vi "Send Command.vi"(6 "Command":T1, 8 "error in":errorcluster, 10 "Value":dbl, 11 "Thorlabs In":refnum<class "Thorlabs.lvclass">) -> (0 "error out":errorcluster, 3 "Thorlabs Out":refnum<class "Thorlabs.lvclass">)   [LabVIEW 2018, in "Thorlabs.lvlib" / "Thorlabs.lvclass"]
doc: "This VI is designed to take in all the possible Commands, and perform the proper functions of that Command. If the Command is not supported nothing happens.\n\nCreator: Slade Jeppesen\nCreated Date: 09/29/20"
uses:
  Thorlabs.lvclass
  PPLs/Axis/Parent/Axis.lvlibp/Custom Controls/Command.ctl
  PPLs/Axis/Parent/Axis.lvlibp
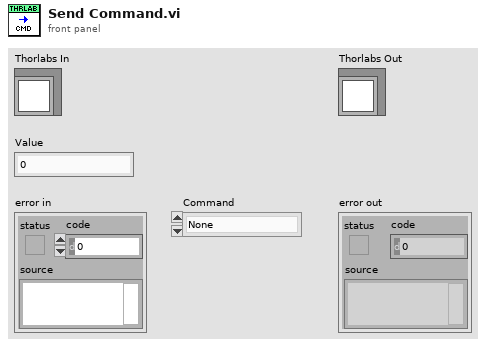
[diagram p1: front panel]
types:
  T1 = typedef "Axis.lvlibp/Command.ctl" = enum16{"None", "Home", "Renumber", "Move Absolute", "Move Relative", "Stop", "Set Run Speed", "Set Acceleration", "Set Run Current", "Set Home Offset", "Set Home Speed", "Query Current Position", "Load Defaults", "Query Status", "Lock Controls", "Unlock Controls", "Set Jog Step Size", "Set Jog Acceleration", "Set Jog Speed", "Query Homed Status", "Query Moving Status", "Reset", "Set Max Position", "Set Min Position"}
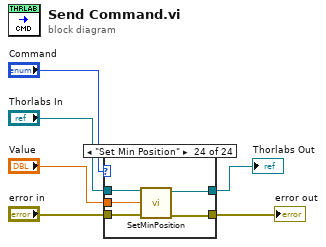
[diagram p0: block diagram]
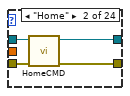
[diagram p3: hidden frame]
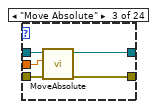
[diagram p4: hidden frame]
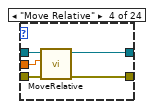
[diagram p5: hidden frame]
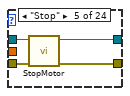
[diagram p6: hidden frame]
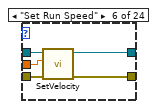
[diagram p7: hidden frame]
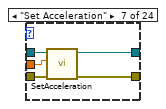
[diagram p8: hidden frame]
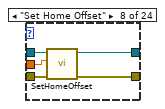
[diagram p9: hidden frame]
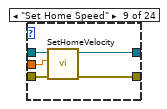
[diagram p10: hidden frame]
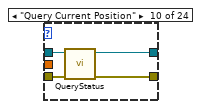
[diagram p11: hidden frame]
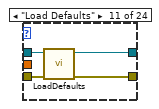
[diagram p12: hidden frame]
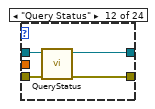
[diagram p13: hidden frame]
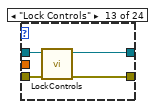
[diagram p14: hidden frame]
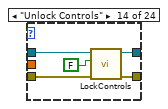
[diagram p15: hidden frame]
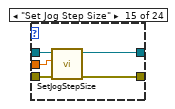
[diagram p16: hidden frame]
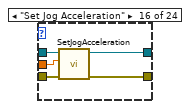
[diagram p17: hidden frame]
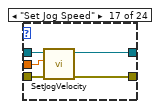
[diagram p18: hidden frame]
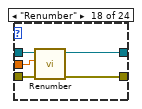
[diagram p19: hidden frame]
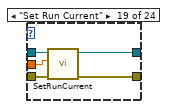
[diagram p20: hidden frame]
diagram:
  n1 = case shown="\"Set Min Position\"" "Command" {
    tunnel: "Value" -> [_ _ w16 w18 _ w30 w35 w40 w44 _ _ _ _ _ w71 w75 w80 w83 w88 _ _ _ w108 w110]
    tunnel: "Thorlabs In" -> [w7 w11 w15 w19 w25 w29 w34 w39 w45 w49 w53 w57 w61 w66 w70 w76 w81 w86 w91 w95 w99 w101 w109 w114]
    tunnel: "error in" -> [w8 w12 w17 w22 w26 w31 w36 w41 w46 w50 w54 w58 w62 w67 w72 w77 w82 w87 w92 w96 w100 w104 w107 w111]
    tunnel: [w8 w9 w13 w21 w23 w27 w32 w37 w42 w47 w51 w55 w59 w63 w68 w73 w78 w84 w89 w93 w97 w103 w106 w112] -> w1
    tunnel: [w7 w10 w14 w20 w24 w28 w33 w38 w43 w48 w52 w56 w60 w65 w69 w74 w79 w85 w90 w94 w98 w102 w105 w113] -> w2
    frame "None", Default {
    }
    frame "Home" {
      n2 = call "HomeCMD.vi"("Error In"=w12, "Thorlabs In"=w11) -> ("Error Out"=w9:errorcluster, "Thorlabs Out"=w10:refnum<class "Thorlabs.lvclass">)  [unwired: 8 in]
    }
    frame "Move Absolute" {
      n3 = call "MoveAbsolute.vi"("Error In"=w17, "Move Abs Value"=w16, "Thorlabs In"=w15) -> ("Error Out"=w13:errorcluster, "Thorlabs Out"=w14:refnum<class "Thorlabs.lvclass">)  [unwired: 7 in]
    }
    frame "Move Relative" {
      n4 = call "MoveRelative.vi"("Error In"=w22, "Move Relative Value"=w18, "Thorlabs In"=w19) -> ("Error Out"=w21:errorcluster, "Thorlabs Out"=w20:refnum<class "Thorlabs.lvclass">)  [unwired: 7 in]
    }
    frame "Stop" {
      n5 = call "StopMotor.vi"("Error In"=w26, "Thorlabs In"=w25) -> ("Error Out"=w23:errorcluster, "Thorlabs Out"=w24:refnum<class "Thorlabs.lvclass">)  [unwired: 8 in]
    }
    frame "Set Run Speed" {
      n6 = call "SetVelocity.vi"("Error In"=w31, "Velocity"=w30, "Thorlabs In"=w29) -> ("Error Out"=w27:errorcluster, "Thorlabs Out"=w28:refnum<class "Thorlabs.lvclass">)  [unwired: 7 in]
    }
    frame "Set Acceleration" {
      n7 = call "SetAcceleration.vi"("Error In"=w36, "Acceleration"=w35, "Thorlabs In"=w34) -> ("Error Out"=w32:errorcluster, "Thorlabs Out"=w33:refnum<class "Thorlabs.lvclass">)  [unwired: 7 in]
    }
    frame "Set Home Offset" {
      n8 = call "SetHomeOffset.vi"("Error In"=w41, "Offset"=w40, "Thorlabs In"=w39) -> ("Error Out"=w37:errorcluster, "Thorlabs Out"=w38:refnum<class "Thorlabs.lvclass">)  [unwired: 7 in]
    }
    frame "Set Home Speed" {
      n9 = call "SetHomeVelocity.vi"("Error In"=w46, "Velocity"=w44, "Thorlabs In"=w45) -> ("Error Out"=w42:errorcluster, "Thorlabs Out"=w43:refnum<class "Thorlabs.lvclass">)  [unwired: 7 in]
    }
    frame "Query Current Position" {
      n10 = call "QueryStatus.vi"("Error In"=w50, "Thorlabs In"=w49) -> ("Error Out"=w47:errorcluster, "Thorlabs Out"=w48:refnum<class "Thorlabs.lvclass">)  [unwired: 8 in]
    }
    frame "Load Defaults" {
      n11 = call "LoadDefaults.vi"("Error In"=w54, "Thorlabs In"=w53) -> ("Error Out"=w51:errorcluster, "Thorlabs Out"=w52:refnum<class "Thorlabs.lvclass">)  [unwired: 8 in]
    }
    frame "Query Status" {
      n12 = call "QueryStatus.vi"("Error In"=w58, "Thorlabs In"=w57) -> ("Error Out"=w55:errorcluster, "Thorlabs Out"=w56:refnum<class "Thorlabs.lvclass">)  [unwired: 8 in]
    }
    frame "Lock Controls" {
      n13 = call "LockControls.vi"("Error In"=w62, "Thorlabs In"=w61) -> ("Error Out"=w59:errorcluster, "Thorlabs Out"=w60:refnum<class "Thorlabs.lvclass">)  [unwired: 8 in]
    }
    frame "Unlock Controls" {
      n14 = call "LockControls.vi"("Error In"=w67, "Lock? (T)"=FALSE, "Thorlabs In"=w66) -> ("Error Out"=w63:errorcluster, "Thorlabs Out"=w65:refnum<class "Thorlabs.lvclass">)  [unwired: 7 in]
    }
    frame "Set Jog Step Size" {
      n15 = call "SetJogStepSize.vi"("Error In"=w72, "Jog Step Size"=w71, "Thorlabs In"=w70) -> ("Error Out"=w68:errorcluster, "Thorlabs Out"=w69:refnum<class "Thorlabs.lvclass">)  [unwired: 7 in]
    }
    frame "Set Jog Acceleration" {
      n16 = call "SetJogAcceleration.vi"("Error In"=w77, "Jog Acceleration"=w75, "Thorlabs In"=w76) -> ("Error Out"=w73:errorcluster, "Thorlabs Out"=w74:refnum<class "Thorlabs.lvclass">)  [unwired: 7 in]
    }
    frame "Set Jog Speed" {
      n17 = call "SetJogVelocity.vi"("Error In"=w82, "Jog Velocity"=w80, "Thorlabs In"=w81) -> ("Error Out"=w78:errorcluster, "Thorlabs Out"=w79:refnum<class "Thorlabs.lvclass">)  [unwired: 7 in]
    }
    frame "Renumber" {
      n18 = call "Renumber.vi"("Error In"=w87, "Value"=w83, "Thorlabs in"=w86) -> ("Error Out"=w84:errorcluster, "Thorlabs out"=w85:refnum<class "Thorlabs.lvclass">)  [unwired: 7 in]
    }
    frame "Set Run Current" {
      n19 = call "SetRunCurrent.vi"("Error In"=w92, "Value"=w88, "Thorlabs in"=w91) -> ("Error Out"=w89:errorcluster, "Thorlabs out"=w90:refnum<class "Thorlabs.lvclass">)  [unwired: 7 in]
    }
    frame "Query Homed Status" {
      n20 = call "QueryStatus.vi"("Error In"=w96, "Thorlabs In"=w95) -> ("Error Out"=w93:errorcluster, "Thorlabs Out"=w94:refnum<class "Thorlabs.lvclass">)  [unwired: 8 in]
    }
    frame "Query Moving Status" {
      n21 = call "QueryStatus.vi"("Error In"=w100, "Thorlabs In"=w99) -> ("Error Out"=w97:errorcluster, "Thorlabs Out"=w98:refnum<class "Thorlabs.lvclass">)  [unwired: 8 in]
    }
    frame "Reset" {
      n22 = call "Reset.vi"("Error In"=w104, "Thorlabs in"=w101) -> ("Error Out"=w103:errorcluster, "Thorlabs out"=w102:refnum<class "Thorlabs.lvclass">)  [unwired: 8 in]
    }
    frame "Set Max Position" {
      n23 = call "SetMaxPosition.vi"("Error In"=w107, "Max Position"=w108, "Thorlabs In"=w109) -> ("Error Out"=w106:errorcluster, "Thorlabs Out"=w105:refnum<class "Thorlabs.lvclass">)  [unwired: 7 in]
    }
    frame "Set Min Position" {
      n24 = call "SetMinPosition.vi"("Error In"=w111, "Min Position"=w110, "Thorlabs In"=w114) -> ("Error Out"=w112:errorcluster, "Thorlabs Out"=w113:refnum<class "Thorlabs.lvclass">)  [unwired: 7 in]
    }
  }
  "error out" <- w1
  "Thorlabs Out" <- w2
